vi "例4.13-3轮询+延时（常见问题8）.vi"() -> ()   [LabVIEW 2017]
panel:
  out "和":dbl
  in  "加数2":dbl
  in  "加数1":dbl
  in  "停止":bool
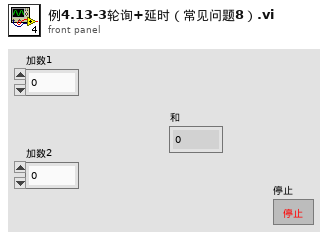
[diagram p1: front panel]
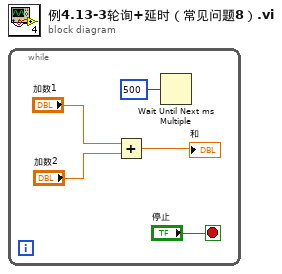
[diagram p0: block diagram]
diagram:
  n1 = while {
    stop <- "停止" stop-if-true
    n2 = Add(x="加数1", y="加数2") -> (x+y=→"和":dbl)
    n3 = Wait Until Next ms Multiple(millisecond multiple=u32 500 ("毫秒倍数")) -> ()  [unwired: 1 out]
  }
